vi "Configure Coupling.vi"(8 "error in (no error)":errorcluster, 10 "Enable Coupling (0:Off)":u16(ring) items=["Off", "Channels 1 & 2", "Channels 2 & 3", "Channels 1 & 3", "All"], 11 "VISA resource name":refnum<visa-resource-name>) -> (0 "error out":errorcluster, 3 "VISA resource name out":refnum<visa-resource-name>)   [LabVIEW 2012, in "BK Precision 913XX.lvlib"]
doc: "Enables or disables coupling for the selected channels."
uses:
  <instrlib>/BK Precision 913XX/BK Precision 913XX.lvlib
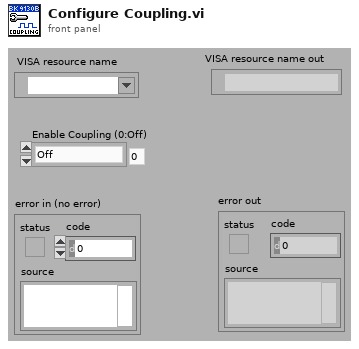
[diagram p1: front panel]
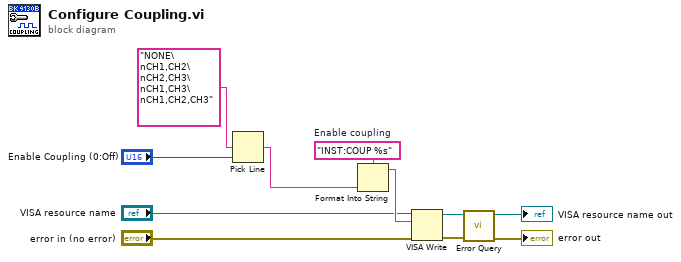
[diagram p0: block diagram]
diagram:
  w7 = "INST:COUP %s"  # Enable coupling
  n1 = Pick Line(multi-line string="NONE\nCH1,CH2\nCH2,CH3\nCH1,CH3\nCH1,CH2,CH3", line index="Enable Coupling (0:Off)") -> (output string=w1:string)  [unwired: 1 in]
  n2 = Format Into String(format string=w7, w1) -> (resulting string=w6:string)  [unwired: 2 in, 1 out]
  n3 = VISA Write(VISA resource name="VISA resource name", write buffer=w6, error in (no error)="error in (no error)") -> (VISA resource name out=w9:refnum<visa-resource-name>, error out=w8:errorcluster)  [unwired: 1 out]
  n4 = call <instrlib>:"Error Query.vi"("error in (no error)"=w8, "VISA resource name"=w9) -> ("error out"=→"error out":errorcluster, "VISA resource name out"=→"VISA resource name out":refnum<visa-resource-name>)  [unwired: 6 in, 2 out]
